vi "conv_temp.vi"(7 "sens_type":T1 caption="Sensor Type" items=["SHTC3", "SHT3X", "D6T_1A", "HTS221", "AHT20", "ADT7410"], 9 "length (rest)":i32, 10 "offset (0)":i32, 11 "Response":string) -> (1 "rh":T2 format="%#_4g", 2 "f_temp":T3 format="%_4g")   [LabVIEW 2013]
uses:
  temp_ind.ctl
  rh_ind.ctl
  sens_type.ctl
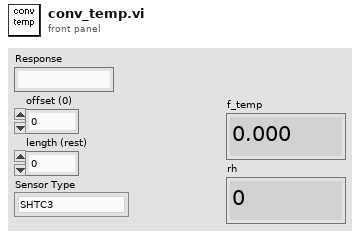
[diagram p1: front panel]
types:
  T1 = typedef "sens_type.ctl" = u8
  T2 = typedef "rh_ind.ctl" = dbl
  T3 = typedef "temp_ind.ctl" = dbl
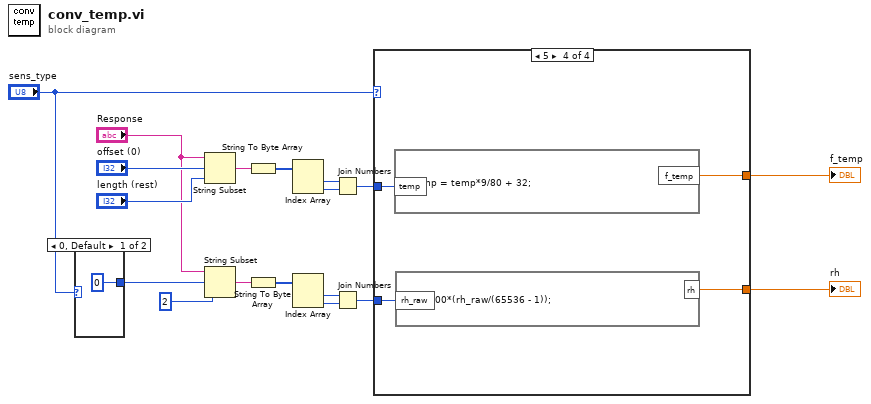
[diagram p0: block diagram]
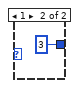
[diagram p2: hidden frame]
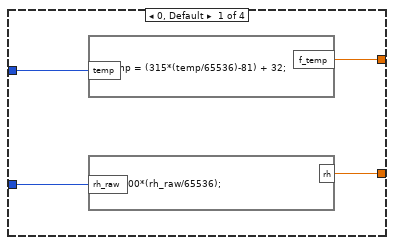
[diagram p3: hidden frame]
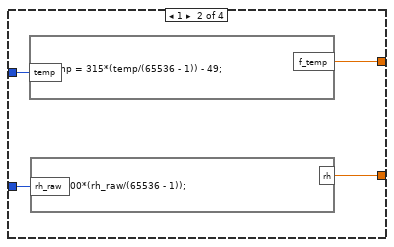
[diagram p4: hidden frame]
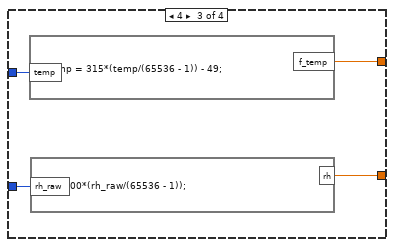
[diagram p5: hidden frame]
diagram:
  n1 = case shown="0, Default" "sens_type" {
    tunnel: [0 ("offset (0)") 3 ("offset (0)")] -> w1
    frame 0, Default {
    }
    frame 1 {
    }
  }
  n2 = String Subset(string="Response", offset (0)="offset (0)", length (rest)="length (rest)") -> (substring=w15:string)
  n3 = String Subset(string="Response", offset (0)=w1, length (rest)=2 ("length (rest)")) -> (substring=w11:string)
  n4 = String To Byte Array(string=w15) -> (unsigned byte array=w16:u8[])
  n5 = String To Byte Array(string=w11) -> (unsigned byte array=w10:u8[])
  n6 = Index Array(array=w16) -> (element #1=w17:u8, element #2=w18:u8)  [unwired: 2 in]
  n7 = Index Array(array=w10) -> (element #1=w7:u8, element #2=w6:u8)  [unwired: 2 in]
  n8 = Join Numbers(hi=w17, lo=w18) -> ((hi.lo)=w12:u16)
  n9 = Join Numbers(hi=w7, lo=w6) -> ((hi.lo)=w5:u16)
  n10 = case shown="5" "sens_type" {
    tunnel: w12 -> [w24 w28 w32 w36]
    tunnel: w5 -> [w23 w27 w31 w35]
    tunnel: [w22 w26 w30 w34] -> w4
    tunnel: [w21 w25 w29 w33] -> w3
    frame 0, Default {
      n11 = formula code="f_temp = (315*(temp/65536)-81) + 32;"("temp"=w24) -> ("f_temp"=w22:dbl)
      n12 = formula code="rh = 100*(rh_raw/65536);"("rh_raw"=w23) -> ("rh"=w21:dbl)
    }
    frame 1 {
      n13 = formula code="f_temp = 315*(temp/(65536 - 1)) - 49;"("temp"=w28) -> ("f_temp"=w26:dbl)
      n14 = formula code="rh = 100*(rh_raw/(65536 - 1));"("rh_raw"=w27) -> ("rh"=w25:dbl)
    }
    frame 4 {
      n15 = formula code="f_temp = 315*(temp/(65536 - 1)) - 49;"("temp"=w32) -> ("f_temp"=w30:dbl)
      n16 = formula code="rh = 100*(rh_raw/(65536 - 1));"("rh_raw"=w31) -> ("rh"=w29:dbl)
    }
    frame 5 {
      n17 = formula code="f_temp = temp*9/80 + 32;"("temp"=w36) -> ("f_temp"=w34:dbl)
      n18 = formula code="rh = 100*(rh_raw/(65536 - 1));"("rh_raw"=w35) -> ("rh"=w33:dbl)
    }
  }
  "f_temp" <- w4
  "rh" <- w3
